vi "NetComm_SetNewDataOccurrenceReference.vi"(8 "error in":errorcluster, 11 "occurrence":refnum<k4>) -> (0 "error out":errorcluster)   [LabVIEW 2017]
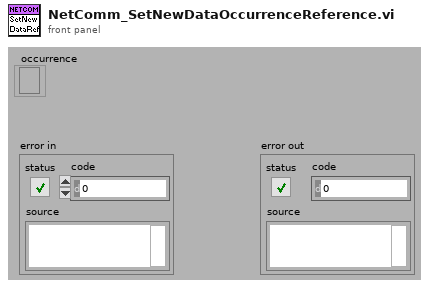
[diagram p1: front panel]
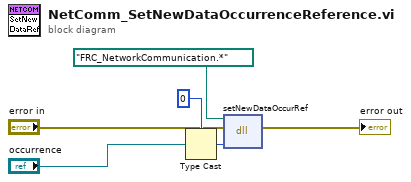
[diagram p0: block diagram]
diagram:
  n1 = Type Cast(type=u32 0 ("element"), x="occurrence") -> (*(type *) &x=w4:u32)
  n2 = dll-call lib="FRC_NetworkCommunication.*" fn="setNewDataOccurRef"(path in=path "FRC_NetworkCommunication.*", error in="error in", "Ref"=w4) -> (error out=→"error out":errorcluster)  [unwired: 2 in, 2 out]
